vi "总磷氨氮通讯.vi"() -> ()   [LabVIEW 2016, in "CodCr.lvlib"]
uses:
  CodCr.lvlib
  <vilib>/Plasmionique/MB Master/MB_Master_Serial/MB_Master_Serial.lvclass
  <vilib>/Utility/config.llb/NI_LVConfig.lvlib
  <vilib>/Plasmionique/MB Master/MB_Master/MB_Master.lvclass
  <vilib>/Plasmionique/MB Master/MB Master.lvlib
  <vilib>/ptbypt/NI_PtbyPt.lvlib
  <vilib>/Utility/config.llb/Write Key (String).vi
  <vilib>/Utility/config.llb/Read Key (String).vi
  <vilib>/Utility/config.llb/Write Key (Boolean).vi
  <vilib>/Utility/config.llb/Read Key (Boolean).vi
  F:/Program Files/National Instruments/LabVIEW 2016/vi.lib/Plasmionique/MB Master/MB_Master/MB_Master.lvclass
panel:
  out "序列号":string
  out "状态告警区":T1
  out "测量数据区":T2 {"单位" items=["ug/L", "mg/L", "ppm", "mg/m3", "cm", "ppb", "ug/m3", "%", "nmol/mol", "umol/mol", "MPN/L", "MPN/100ml", "ng/m3", "NTU", "无量纲", "ms/cm", "us/cm", "℃", "mV", "万个/L"]}
  out "status":bool
  out "关键参数区":T3
  in  "读关键参数区":bool
  in  "读状态告警区":bool
  in  "读测量数据区":bool
  in  "站号":u16(ring) items=["总磷"=1, "氨氮"=3]
  in  "停止":bool
  in  "启动":bool
  in  "控制命令":u16(ring) items=["启动测量"=1, "标样核查"=2, "零点核查"=3, "跨度核查"=4, "空白测试"=5, "平行样测试"=6, "加标回收"=7, "空白校准"=8, "标样校准"=9, "初始化（清洗）"=10, "停止测试"=11, "仪器重启"=12, "校时"=13, "模式设置"=14, "测量间隔设置"=15]
  in  "控制命令参数":u16[](array[numeric]) format="%04xH"
  in  "VISA Resource":refnum<visa-resource-name>="COM16"
  in  "启用模块":bool
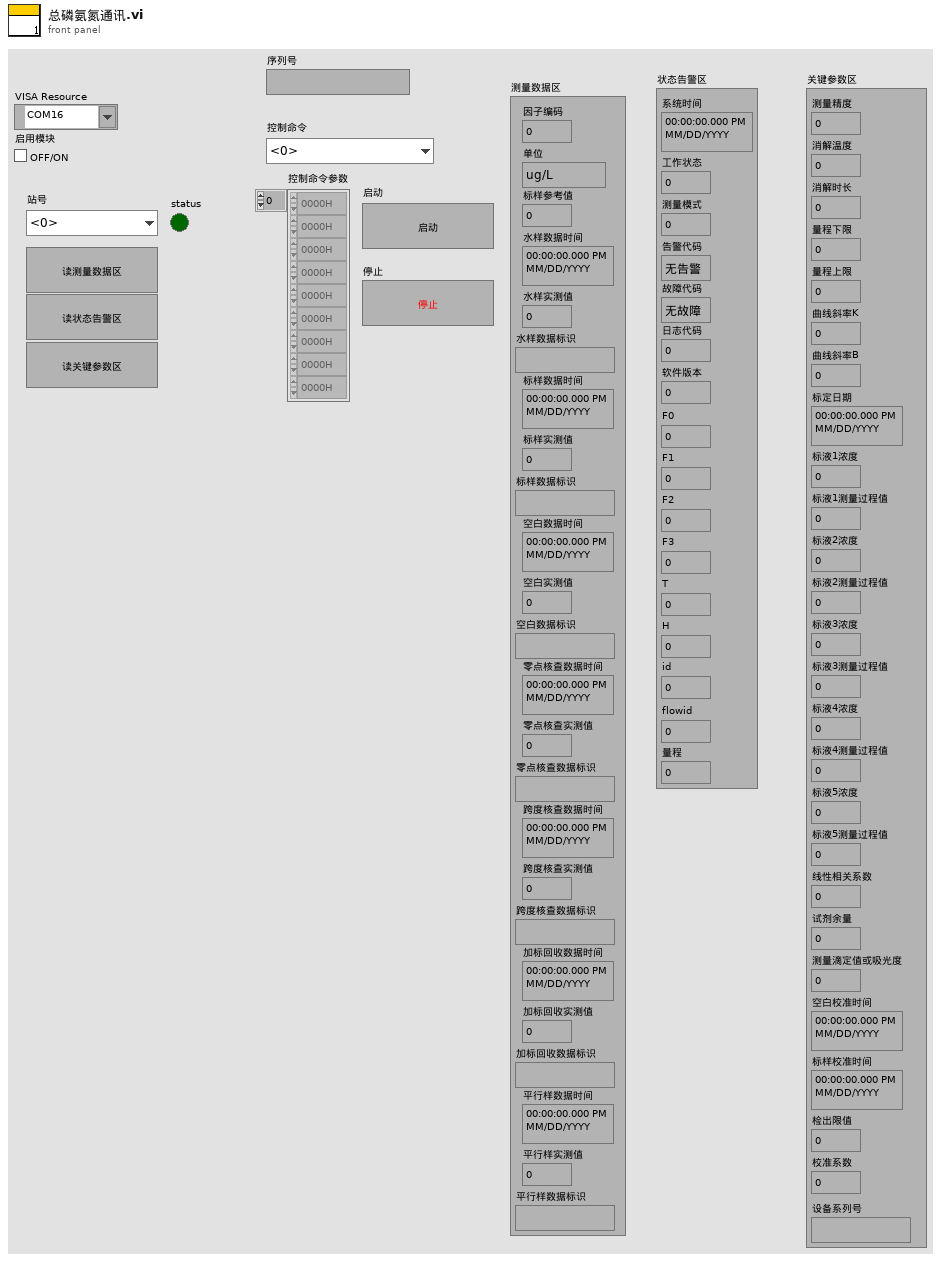
[diagram p1: front panel]
types:
  T1 = cluster{"系统时间":timestamp, "工作状态":u16, "测量模式":u16, "告警代码":enum16{"无告警", "缺试剂告警", "缺水样告警", "缺蒸馏水告警", "缺标液告警", "仪表漏液告警", "标定异常告警", "超量程告警", "加热异常", "低试剂预警", "超上限告警", "超下限告警", "仪表内部其他异常", "滴定异常告警", "电极异常告警", "量程切换告警", "参数设置告警", "PH电极电位异常", "电导率电极异常", "浊度光度异常", "溶解氧电极异常", "溶解氧光强异常", "温度异常告警", "PH异常告警", "溶解氧异常告警", "电导率异常告警", "浊度异常告警", "叶绿素异常告警", "藻密度异常告警", "蓝绿藻异常告警", "ORP异常告警", "氨氮异常告警", "清洁刷异常告警", "SD卡异常告警", "蓝牙异常告警", "Wifi异常告警", "流程异常告警"}, "故障代码":enum16{"无故障", "电机故障", "温度故障", "通讯故障", "滴定故障"}, "日志代码":u16, "软件版本":u16, "F0":sgl, "F1":sgl, "F2":sgl, "F3":sgl, "T":sgl, "H":sgl, "id":u16, "flowid":u16, "量程":u16}
  T2 = cluster{"因子编码":u32, "单位":u16, "标样参考值":sgl, "水样数据时间":timestamp, "水样实测值":sgl, "水样数据标识":string, "标样数据时间":timestamp, "标样实测值":sgl, "标样数据标识":string, "空白数据时间":timestamp, "空白实测值":sgl, "空白数据标识":string, "零点核查数据时间":timestamp, "零点核查实测值":sgl, "零点核查数据标识":string, "跨度核查数据时间":timestamp, "跨度核查实测值":sgl, "跨度核查数据标识":string, "加标回收数据时间":timestamp, "加标回收实测值":sgl, "加标回收数据标识":string, "平行样数据时间":timestamp, "平行样实测值":sgl, "平行样数据标识":string}
  T3 = cluster{"测量精度":u16, "消解温度":u16, "消解时长":u16, "量程下限":sgl, "量程上限":sgl, "曲线斜率K":sgl, "曲线斜率B":sgl, "标定日期":timestamp, "标液1浓度":sgl, "标液1测量过程值":sgl, "标液2浓度":sgl, "标液2测量过程值":sgl, "标液3浓度":sgl, "标液3测量过程值":sgl, "标液4浓度":sgl, "标液4测量过程值":sgl, "标液5浓度":sgl, "标液5测量过程值":sgl, "线性相关系数":sgl, "试剂余量":u32, "测量滴定值或吸光度":sgl, "空白校准时间":timestamp, "标样校准时间":timestamp, "检出限值":sgl, "校准系数":sgl, "设备系列号":string}
  T4 = typedef "NI_LVConfig.lvlib/Config Data RefNum.ctl" = refnum<k1>
  T5 = enum8{"Enabled", "Disabled", "Disabled and Grayed Out"}
  T6 = cluster{"baud rate (bps)":u32, "stop bits":u16, "parity":u16, "flow control":u16, "timeout":u32, "retries":i32}
  T7 = cluster{"因子编码":u32, "单位":u16, "标样参考值":sgl, "水样数据时间":timestamp, "水样实测值":sgl, "水样数据标识":string, "标样数据时间":timestamp, "标样实测值":sgl, "标样数据标识":string, "空白数据时间":timestamp, "空白实测值":sgl, "空白数据标识":string, "零点核查数据时间":timestamp, "零点核查实测值":sgl, "零点核查数据标识":string, "跨度核查数据时间":timestamp, "跨度核查实测值":sgl, "跨度核查数据标识":string, "加标回收数据时间":timestamp, "加标回收实测值":sgl, "加标回收数据标识":string, "平行样数据时间":timestamp, "平行样实测值":sgl, "平行样数据标识":string, "F0":sgl, "F1":sgl, "F2":sgl, "F3":sgl, "F4":sgl, "F5":sgl, "F6":sgl, "F7":sgl, "温度":sgl, "湿度":sgl, "X值":sgl}
  T8 = cluster{"系统时间":timestamp, "工作状态":enum16{"空闲", "水样测试", "标样核查", "零点核查", "跨度核查", "空白测试", "平行样测试", "加标回收", "空白校准", "标样校准", "初始化（清洗）"}, "测量模式":enum16{"待机", "连续模式", "周期模式", "定点模式", "受控模式", "手动模式"}, "告警代码":enum16{"无告警", "缺试剂告警", "缺水样告警", "缺蒸馏水告警", "缺标液告警", "仪表漏液告警", "标定异常告警", "超量程告警", "加热异常", "低试剂预警", "超上限告警", "超下限告警", "仪表内部其他异常", "滴定异常告警", "电极异常告警", "量程切换告警", "参数设置告警", "PH电极电位异常", "电导率电极异常", "浊度光度异常", "溶解氧电极异常", "溶解氧光强异常", "温度异常告警", "PH异常告警", "溶解氧异常告警", "电导率异常告警", "浊度异常告警", "叶绿素异常告警", "藻密度异常告警", "蓝绿藻异常告警", "ORP异常告警", "氨氮异常告警", "清洁刷异常告警", "SD卡异常告警", "蓝牙异常告警", "Wifi异常告警", "流程异常告警"}, "故障代码":enum16{"无故障", "电机故障", "温度故障", "通讯故障", "滴定故障"}, "日志代码":u16, "软件版本":u16, "F0":sgl, "F1":sgl, "F2":sgl, "F3":sgl, "T":sgl, "H":sgl, "id":u16, "flowid":u16, "量程":u16, "总磷控温温度1":sgl, "营养盐控温温度2":sgl, "ADC":sgl}
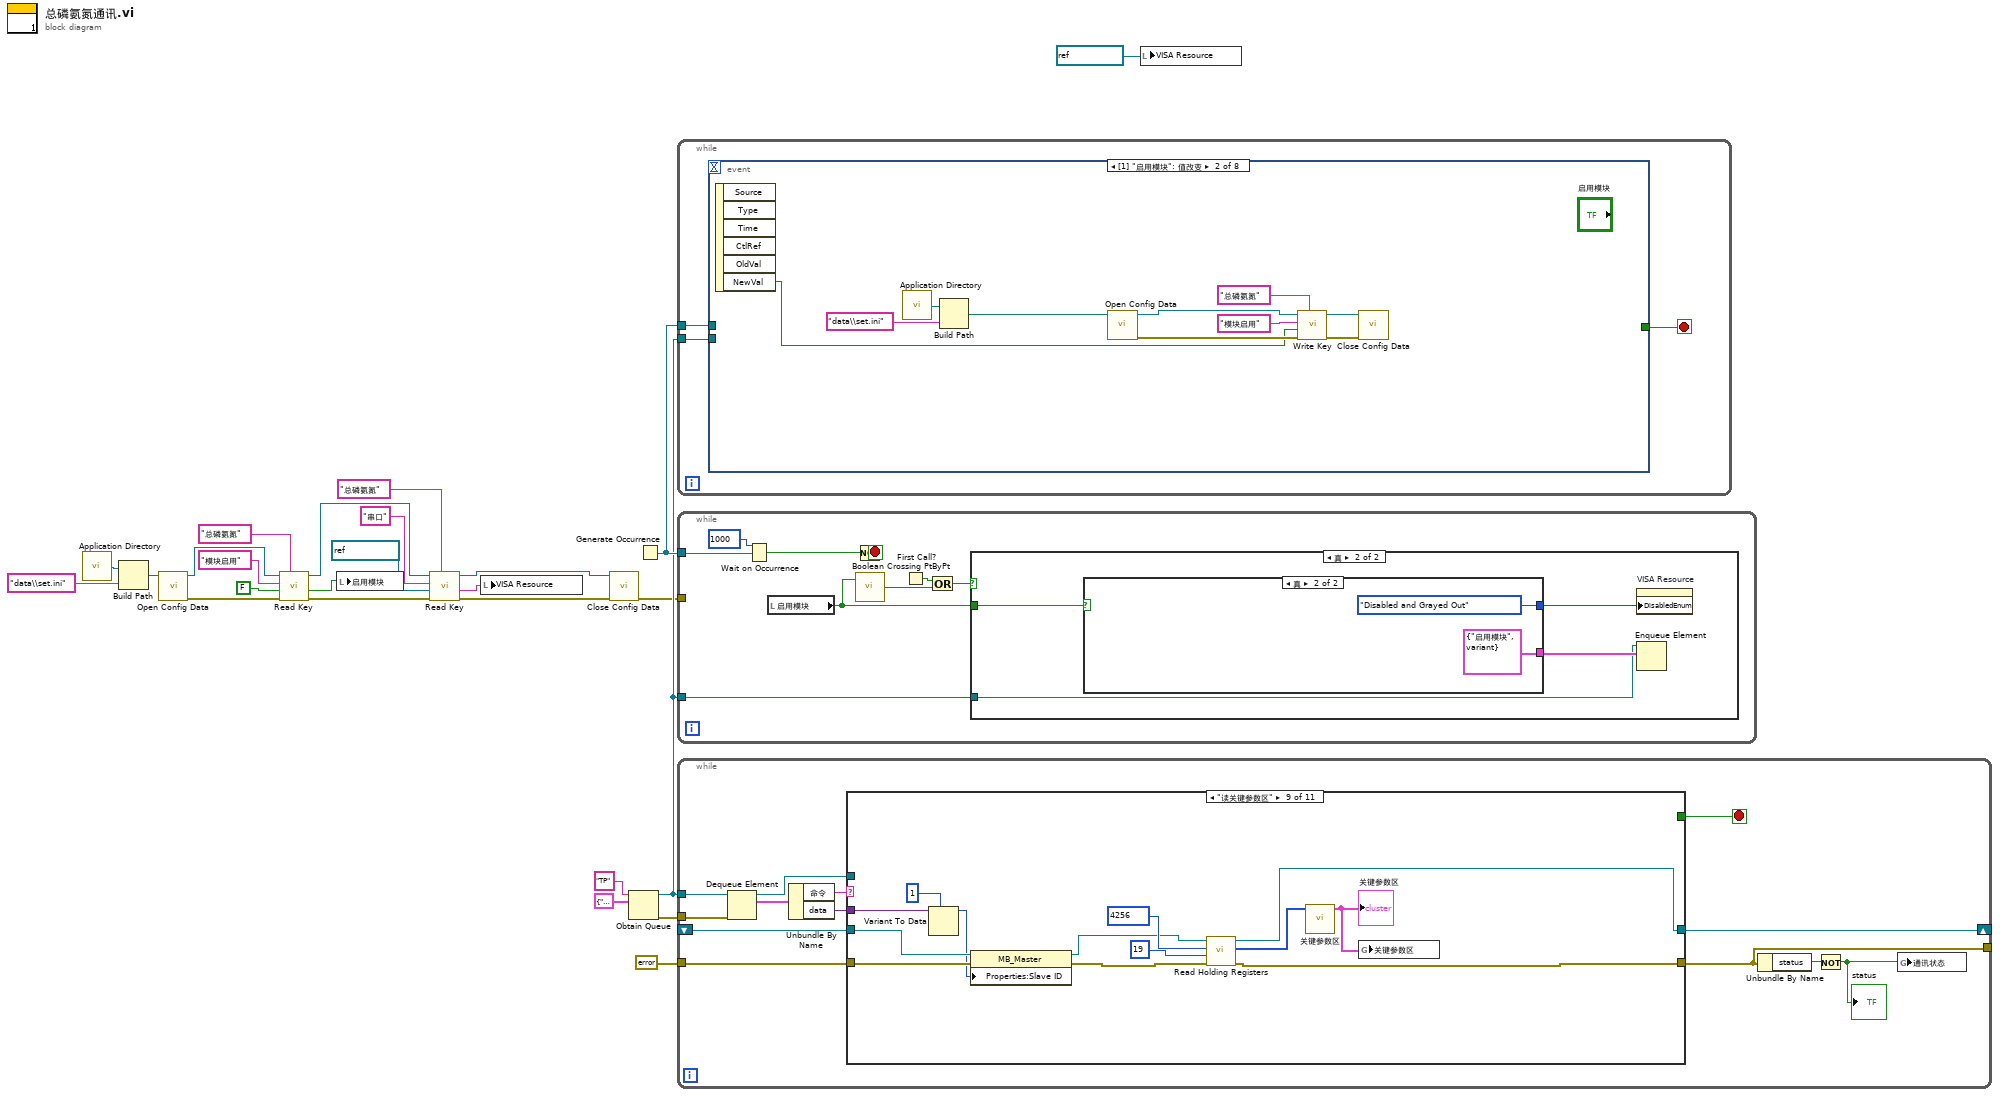
[diagram p0: block diagram]
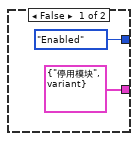
[diagram p3: hidden frame]
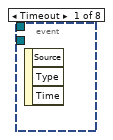
[diagram p4: hidden frame]
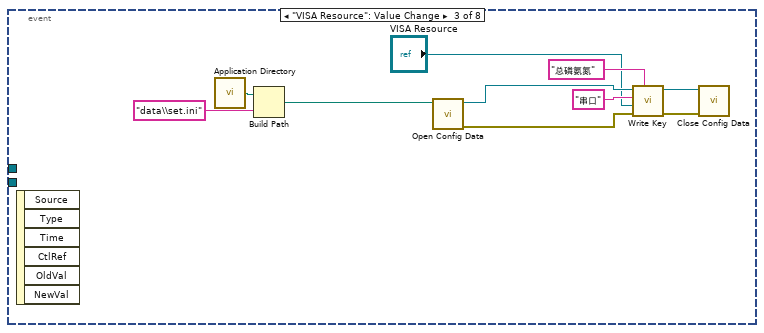
[diagram p5: hidden frame]
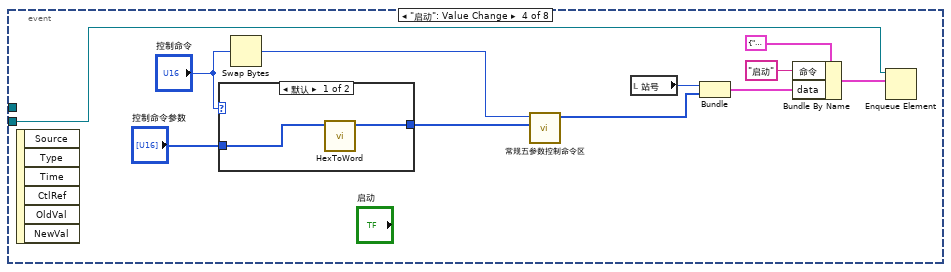
[diagram p6: hidden frame]
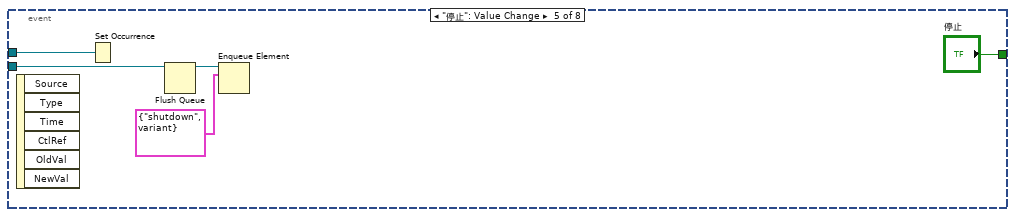
[diagram p8: hidden frame]
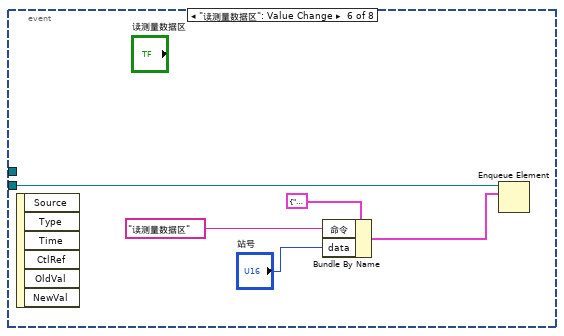
[diagram p9: hidden frame]
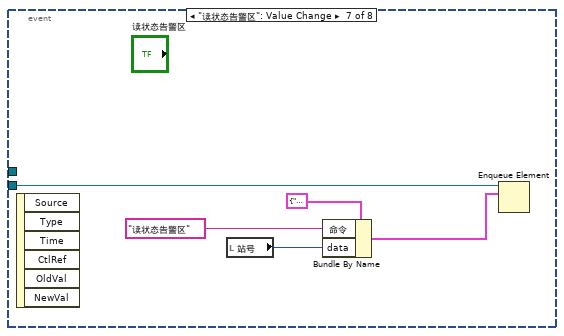
[diagram p10: hidden frame]
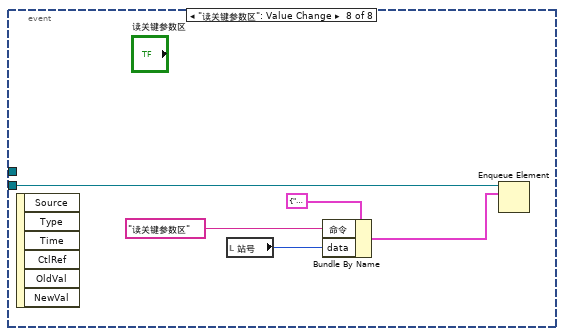
[diagram p11: hidden frame]
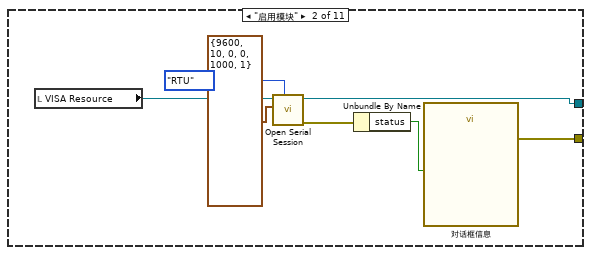
[diagram p13: hidden frame]
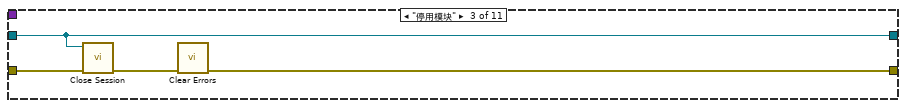
[diagram p14: hidden frame]
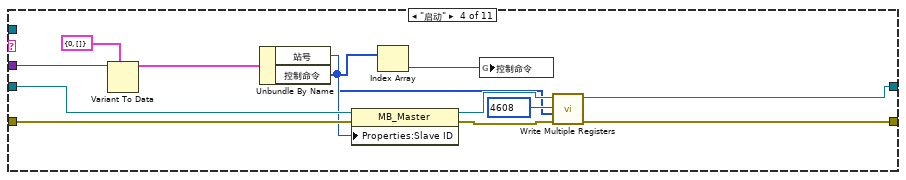
[diagram p15: hidden frame]
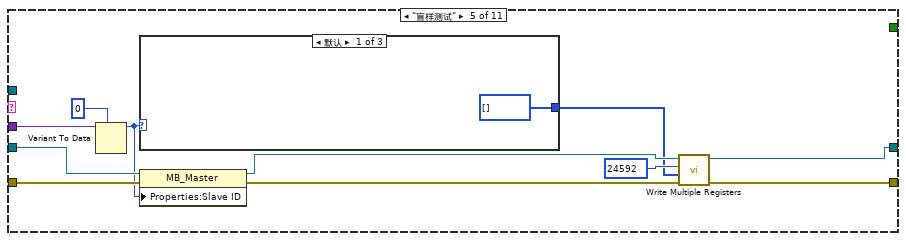
[diagram p16: hidden frame]
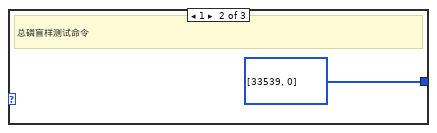
[diagram p17: hidden frame]
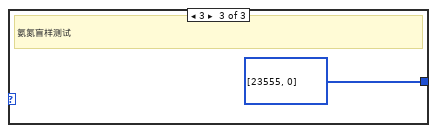
[diagram p18: hidden frame]
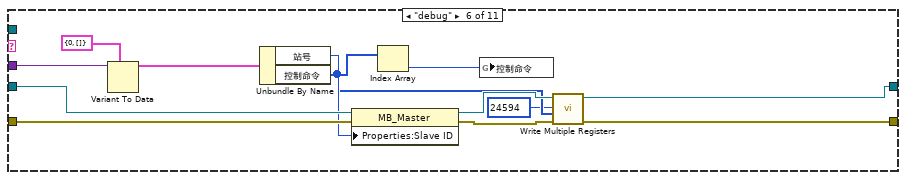
[diagram p19: hidden frame]
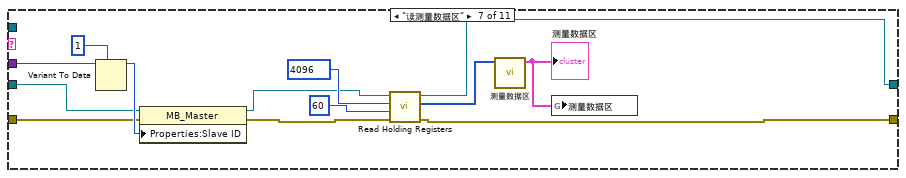
[diagram p20: hidden frame]
diagram:
  n1 = call <vilib>:"Application Directory.vi"() -> ("Application Directory"=w13:path)
  n2 = Build Path(base path=w13, name or relative path="data\\set.ini" ("名称或相对路径")) -> (appended path=w14:path)
  n3 = call <vilib>:"Open Config Data.vi"("configuration file path"=w14) -> ("error out"=w19:errorcluster, "refnum"=w18:T4)  [unwired: 8 in, 1 out]
  n4 = call-poly <vilib>:"Read Key.vi"("section"="总磷氨氮", "error in (no error)"=w19, "default value"=FALSE ("启用模块"), "key"="模块启用", "refnum"=w18) -> ("error out"=w7:errorcluster, "value"=w10:bool, "refnum out"=w9:T4)  [unwired: 3 in, 1 out]
  n5 = local write "启用模块"(w10) -> ()
  n6 = call-poly <vilib>:"Read Key.vi"("section"="总磷氨氮", "error in (no error)"=w7, "default value"=refnum<visa-resource-name> "COM16" ("VISA Resource"), "key"="串口", "refnum"=w9) -> ("error out"=w6:errorcluster, "value"=w3:string, "refnum out"=w8:T4)  [unwired: 3 in, 1 out]
  n7 = local write "VISA Resource"(w3) -> ()
  n8 = call <vilib>:"Close Config Data.vi"("error in (no error)"=w6, "refnum"=w8) -> ("error out"=w11:errorcluster)  [unwired: 8 in, 1 out]
  n9 = Obtain Queue(name (unnamed)="TP" ("名称（未命名）"), element data type=cluster{"命令":string, "data":variant} {"命令"="", "data"=variant}) -> (queue out=w20:refnum<queue>, error out=w23:errorcluster)  [unwired: 3 in, 1 out]
  n10 = Generate Occurrence() -> (w21:refnum<k4>)
  n11 = while {
    tunnel: w20 -> [w28]
    tunnel: w21 -> [w26]
    stop <- w27 stop-if-true
    n12 = event shown="[1] \"启用模块\": 值改变" {
      selector: _ -> [_ _ _ _ _ _ _ _]
      dyn-events: _ -> [_ _ _ _ _ _ _ _]
      timeout: _ -> [_ _ _ _ _ _ _ _]
      tunnel: w28 -> [_ _ _ w59 w66 w72 w77 w82]
      tunnel: [_ _ _ _ "停止" _ _ _] -> w27
      tunnel: w26 -> [_ _ _ _ w63 _ _ _]
      event Timeout {
        n13 = event-data() -> ()  [unwired: 1 in, 3 out]
      }
      event "启用模块": Value Change {
        n14 = event-data() -> ("NewVal"=w29:bool)  [unwired: 1 in, 5 out]
        n15 = call <vilib>:"Application Directory.vi"() -> ("Application Directory"=w31:path)
        n16 = Build Path(base path=w31, name or relative path="data\\set.ini" ("名称或相对路径")) -> (appended path=w32:path)
        n17 = call <vilib>:"Open Config Data.vi"("configuration file path"=w32) -> ("error out"=w38:errorcluster, "refnum"=w37:T4)  [unwired: 8 in, 1 out]
        n18 = call-poly <vilib>:"Write Key.vi"("section"="总磷氨氮", "error in (no error)"=w38, "value"=w29, "key"="模块启用", "refnum"=w37) -> ("error out"=w34:errorcluster, "refnum out"=w30:T4)  [unwired: 4 in, 1 out]
        n19 = call <vilib>:"Close Config Data.vi"("error in (no error)"=w34, "refnum"=w30) -> ()  [unwired: 8 in, 2 out]
      }
      event "VISA Resource": Value Change {
        n20 = event-data() -> ()  [unwired: 1 in, 6 out]
        n21 = call <vilib>:"Application Directory.vi"() -> ("Application Directory"=w41:path)
        n22 = Build Path(base path=w41, name or relative path="data\\set.ini" ("名称或相对路径")) -> (appended path=w42:path)
        n23 = call <vilib>:"Open Config Data.vi"("configuration file path"=w42) -> ("error out"=w48:errorcluster, "refnum"=w47:T4)  [unwired: 8 in, 1 out]
        n24 = call-poly <vilib>:"Write Key.vi"("section"="总磷氨氮", "error in (no error)"=w48, "value"="VISA Resource", "key"="串口", "refnum"=w47) -> ("error out"=w44:errorcluster, "refnum out"=w40:T4)  [unwired: 4 in, 1 out]
        n25 = call <vilib>:"Close Config Data.vi"("error in (no error)"=w44, "refnum"=w40) -> ()  [unwired: 8 in, 2 out]
      }
      event "启动": Value Change {
        n26 = event-data() -> ()  [unwired: 1 in, 6 out]
        n27 = case shown="默认" "控制命令" {
          tunnel: "控制命令参数" -> [w61 w62]
          tunnel: [w60 w62] -> w49
          frame Default {
            n28 = call "HexToWord.vi"("数组"=w61) -> ("WORD"=w60:u16[])  [unwired: 10 in]
          }
          frame 13 {
          }
        }
        n29 = Swap Bytes(anything="控制命令") -> (byte swapped=w52:u16)
        n30 = call "常规五参数控制命令区.vi"("控制命令参数"=w49, "控制命令"=w52) -> ("控制命令输出"=w55:u16[])  [unwired: 9 in]
        n31 = local read "站号"() -> (w54:u16)
        n32 = Bundle("站号"=w54, "控制命令输出"=w55) -> (w53:cluster{"站号":u16, "控制命令输出":u16[]})  [unwired: 1 in]
        n33 = Bundle By Name(cluster=cluster{"命令":string, "data":variant} {"命令"="", "data"=variant} ("元素"), "命令"="启动", "data"=w53) -> (w57:cluster{"命令":string, "data":variant})
        n34 = Enqueue Element(queue=w59, element=w57) -> ()  [unwired: 2 in, 3 out]
      }
      event "停止": Value Change {
        n35 = event-data() -> ()  [unwired: 1 in, 6 out]
        n36 = Set Occurrence(w63) -> ()
        n37 = Flush Queue(queue=w66) -> (queue out=w65:refnum<queue>)  [unwired: 1 in, 2 out]
        n38 = Enqueue Element(queue=w65, element=cluster{"命令":string, "data":variant} {"命令"="shutdown", "data"=variant} ("元素")) -> ()  [unwired: 2 in, 3 out]
      }
      event "读测量数据区": Value Change {
        n39 = event-data() -> ()  [unwired: 1 in, 6 out]
        n40 = Bundle By Name(cluster=cluster{"命令":string, "data":variant} {"命令"="", "data"=variant} ("元素"), "命令"="读测量数据区", "data"="站号") -> (w70:cluster{"命令":string, "data":variant})
        n41 = Enqueue Element(queue=w72, element=w70) -> ()  [unwired: 2 in, 3 out]
      }
      event "读状态告警区": Value Change {
        n42 = event-data() -> ()  [unwired: 1 in, 6 out]
        n43 = local read "站号"() -> (w73:u16)
        n44 = Bundle By Name(cluster=cluster{"命令":string, "data":variant} {"命令"="", "data"=variant} ("元素"), "命令"="读状态告警区", "data"=w73) -> (w75:cluster{"命令":string, "data":variant})
        n45 = Enqueue Element(queue=w77, element=w75) -> ()  [unwired: 2 in, 3 out]
      }
      event "读关键参数区": Value Change {
        n46 = event-data() -> ()  [unwired: 1 in, 6 out]
        n47 = local read "站号"() -> (w78:u16)
        n48 = Bundle By Name(cluster=cluster{"命令":string, "data":variant} {"命令"="", "data"=variant} ("元素"), "命令"="读关键参数区", "data"=w78) -> (w80:cluster{"命令":string, "data":variant})
        n49 = Enqueue Element(queue=w82, element=w80) -> ()  [unwired: 2 in, 3 out]
      }
    }
  }
  n50 = while {
    tunnel: w21 -> [w91]
    tunnel: w20 -> [w86]
    tunnel: w11 -> [_]
    stop <- w88 stop-if-true
    n51 = Wait on Occurrence(2:w91, 3:1000 ("毫秒超时(-1)")) -> (0:w89:bool)  [unwired: 1 in]
    n52 = local read "启用模块"() -> (w87:bool)
    n53 = Not(x=w89) -> (.not. x?=w88:bool)
    n54 = call <vilib>:"Boolean Crossing PtByPt.vi"("input"=w87) -> ("crossing"=w84:bool)  [unwired: 2 in]
    n55 = First Call?() -> (First Call?: T/F=w85:bool)
    n56 = Or(x=w85, y=w84) -> (x .or. y?=w83:bool)
    n57 = case shown="真" w83 {
      tunnel: w87 -> [_ w94]
      tunnel: w86 -> [_ w93]
      frame False {
      }
      frame True {
        n58 = case shown="真" w94 {
          tunnel: [cluster{"命令":string, "data":variant} {"命令"="停用模块", "data"=variant} ("元素") cluster{"命令":string, "data":variant} {"命令"="启用模块", "data"=variant} ("元素")] -> w95
          tunnel: [T5."Enabled" ("禁用") T5."Disabled and Grayed Out" ("禁用")] -> w92
          frame False {
          }
          frame True {
          }
        }
        n59 = property on="VISA Resource" class="VISAName"("DisabledEnum"=w92) -> ()  [unwired: 2 in, 2 out]
        n60 = Enqueue Element(queue=w93, element=w95) -> ()  [unwired: 2 in, 3 out]
      }
    }
  }
  n61 = while {
    tunnel: w20 -> [w112]
    tunnel: w23 -> [w111]
    shift-right: [w109] -> _
    shift-left: _ -> [w108]
    tunnel: errorcluster {"status"=FALSE, "code"=0, "source"=""} ("error out") -> [w107]
    tunnel: [w102] -> _
    stop <- w110 stop-if-true
    n62 = Dequeue Element(queue=w112, error in (no error)=w111) -> (queue out=w103:refnum<queue>, element=w105:cluster{"命令":string, "data":variant})  [unwired: 1 in, 2 out]
    n63 = Unbundle By Name(w105) -> ("命令"=w106:string, "data"=w104:variant)
    n64 = case shown="\"读关键参数区\"" w106 {
      tunnel: w104 -> [_ _ _ w135 w146 w163 w172 w181 w196 w210 _]
      tunnel: w103 -> [_ _ _ _ _ _ _ _ _ _ w223]
      tunnel: [_ _ _ _ _ _ _ _ _ _ TRUE] -> w110
      tunnel: [w113 w121 w122 w138 w149 w165 w177 w190 w203 w217 w219] -> w109
      tunnel: [w114 w116 w123 w137 w148 w164 w178 w191 w204 w218 w220] -> w102
      tunnel: w108 -> [w113 _ w122 w134 w145 w162 w171 w184 w199 w213 w219]
      tunnel: w107 -> [w114 _ w125 w131 w142 w159 w169 w185 w200 w214 w221]
      frame Default {
      }
      frame "启用模块" {
        n65 = local read "VISA Resource"() -> (w115:refnum<visa-resource-name>)
        n66 = call <vilib>:"Open Serial Session.vi"("Mode (RTU)"=enum16{"RTU", "ASCII"}."RTU", "Serial Config"=T6 {"baud rate (bps)"=9600, "stop bits"=10, "parity"=0, "flow control"=0, "timeout"=1000, "retries"=1}, "VISA Resource"=w115) -> ("Error out"=w117:errorcluster, "MB_Serial session"=w121:refnum<class "MB_Master_Serial.lvclass">)  [unwired: 7 in]
        n67 = Unbundle By Name(w117) -> ("status"=w118:bool)
        n68 = call "对话框信息"("Enable"=w118) -> ("error out"=w116:errorcluster)  [unwired: 9 in, 1 out]
      }
      frame "停用模块" {
        n69 = call-dynamic "Close Session.vi"("error in (no error)"=w125, "MB session in"=w122) -> ("error out"=w124:errorcluster)  [unwired: 9 in]
        n70 = call <vilib>:"Clear Errors.vi"("error in (no error)"=w124) -> ("error out"=w123:errorcluster)  [unwired: 5 in, 1 out]
      }
      frame "启动" {
        n71 = Variant To Data(type=cluster{"站号":u16, "控制命令":u16[]} {"站号"=0, "控制命令"=[]} ("输出簇"), Variant=w135) -> (data=w129:cluster{"站号":u16, "控制命令":u16[]})  [unwired: 1 in, 1 out]
        n72 = Unbundle By Name(w129) -> ("站号"=w128:u16, "控制命令"=w126:u16[])
        n73 = property class="MB_Master"(reference=w134, error in=w131, "Properties:Slave ID"=w128) -> (reference out=w133:refnum<class "MB_Master.lvclass">, error out=w132:errorcluster)
        n74 = Index Array(array=w126) -> (element=w127:u16)  [unwired: 1 in]
        n75 = global write "VAR总磷总氮全局变量.vi" "控制命令"(w127) -> ()
        n76 = call <vilib>:"Write Multiple Registers.vi"("error in (no error)"=w132, "values"=w126, "starting address"=u16 4608, "MB session in"=w133) -> ("error out"=w137:errorcluster, "MB session out"=w138:refnum<class "MB_Master.lvclass">)  [unwired: 6 in]
      }
      frame "盲样测试" {
        n77 = Variant To Data(type=0, Variant=w146) -> (data=w139:i32)  [unwired: 1 in, 1 out]
        n78 = case shown="默认" w139 {
          tunnel: [u16[] [] ("values") u16[] [33539, 0] ("values") u16[] [23555, 0] ("values")] -> w141
          frame Default {
          }
          frame 1 {
            # "总磷盲样测试命令"
          }
          frame 3 {
            # "氨氮盲样测试"
          }
        }
        n79 = property class="MB_Master"(reference=w145, error in=w142, "Properties:Slave ID"=w139) -> (reference out=w144:refnum<class "MB_Master.lvclass">, error out=w143:errorcluster)
        n80 = call <vilib>:"Write Multiple Registers.vi"("error in (no error)"=w143, "values"=w141, "starting address"=u16 24592, "MB session in"=w144) -> ("error out"=w148:errorcluster, "MB session out"=w149:refnum<class "MB_Master.lvclass">)  [unwired: 6 in]
      }
      frame "debug" {
        n81 = Variant To Data(type=cluster{"站号":u16, "控制命令":u16[]} {"站号"=0, "控制命令"=[]} ("输出簇"), Variant=w163) -> (data=w157:cluster{"站号":u16, "控制命令":u16[]})  [unwired: 1 in, 1 out]
        n82 = Unbundle By Name(w157) -> ("站号"=w156:u16, "控制命令"=w154:u16[])
        n83 = property class="MB_Master"(reference=w162, error in=w159, "Properties:Slave ID"=w156) -> (reference out=w161:refnum<class "MB_Master.lvclass">, error out=w160:errorcluster)
        n84 = Index Array(array=w154) -> (element=w155:u16)  [unwired: 1 in]
        n85 = global write "VAR总磷总氮全局变量.vi" "控制命令"(w155) -> ()
        n86 = call <vilib>:"Write Multiple Registers.vi"("error in (no error)"=w160, "values"=w154, "starting address"=u16 24594, "MB session in"=w161) -> ("error out"=w164:errorcluster, "MB session out"=w165:refnum<class "MB_Master.lvclass">)  [unwired: 6 in]
      }
      frame "读测量数据区" {
        n87 = Variant To Data(type=u8 1 ("Slave ID"), Variant=w172) -> (data=w173:u8)  [unwired: 1 in, 1 out]
        n88 = property class="MB_Master"(reference=w171, error in=w169, "Properties:Slave ID"=w173) -> (reference out=w170:refnum<class "MB_Master.lvclass">, error out=w168:errorcluster)
        n89 = call <vilib>:"Read Holding Registers.vi"("error in (no error)"=w168, "quantity"=u16 60, "starting address"=u16 4096, "MB session in"=w170) -> ("error out"=w178:errorcluster, "Registers"=w167:u16[], "MB session out"=w177:refnum<class "MB_Master.lvclass">)  [unwired: 5 in]
        n90 = call "测量数据区.vi"("数组"=w167) -> ("测量数据区"=w166:T7)  [unwired: 10 in]
        "测量数据区" <- w166
        n91 = global write "VAR总磷总氮全局变量.vi" "测量数据区"(w166) -> ()
      }
      frame "读状态告警区" {
        n92 = Variant To Data(type=u8 1 ("Slave ID"), Variant=w181) -> (data=w186:u8)  [unwired: 1 in, 1 out]
        n93 = property class="MB_Master"(reference=w184, error in=w185, "Properties:Slave ID"=w186) -> (reference out=w183:refnum<class "MB_Master.lvclass">, error out=w182:errorcluster)
        n94 = call <vilib>:"Read Holding Registers.vi"("error in (no error)"=w182, "quantity"=u16 24, "starting address"=u16 4224, "MB session in"=w183) -> ("error out"=w191:errorcluster, "Registers"=w180:u16[], "MB session out"=w190:refnum<class "MB_Master.lvclass">)  [unwired: 5 in]
        n95 = call "状态告警区.vi"("数组"=w180) -> ("状态告警区"=w179:T8)  [unwired: 10 in]
        "状态告警区" <- w179
        n96 = global write "VAR总磷总氮全局变量.vi" "状态告警区"(w179) -> ()
      }
      frame "读关键参数区" {
        n97 = Variant To Data(type=u8 1 ("Slave ID"), Variant=w196) -> (data=w194:u8)  [unwired: 1 in, 1 out]
        n98 = property class="MB_Master"(reference=w199, error in=w200, "Properties:Slave ID"=w194) -> (reference out=w198:refnum<class "MB_Master.lvclass">, error out=w197:errorcluster)
        n99 = call <vilib>:"Read Holding Registers.vi"("error in (no error)"=w197, "quantity"=u16 19, "starting address"=u16 4256, "MB session in"=w198) -> ("error out"=w204:errorcluster, "Registers"=w193:u16[], "MB session out"=w203:refnum<class "MB_Master.lvclass">)  [unwired: 5 in]
        n100 = call "关键参数区.vi"("数组"=w193) -> ("关键参数区"=w192:T3)  [unwired: 10 in]
        "关键参数区" <- w192
        n101 = global write "VAR总磷总氮全局变量.vi" "关键参数区"(w192) -> ()
      }
      frame "读序列号" {
        n102 = Variant To Data(type=u8 1 ("Slave ID"), Variant=w210) -> (data=w208:u8)  [unwired: 1 in, 1 out]
        n103 = property class="MB_Master"(reference=w213, error in=w214, "Properties:Slave ID"=w208) -> (reference out=w212:refnum<class "MB_Master.lvclass">, error out=w211:errorcluster)
        n104 = call <vilib>:"Read Holding Registers.vi"("error in (no error)"=w211, "quantity"=u16 6, "starting address"=u16 3, "MB session in"=w212) -> ("error out"=w218:errorcluster, "Registers"=w207:u16[], "MB session out"=w217:refnum<class "MB_Master.lvclass">)  [unwired: 5 in]
        n105 = call "HexToString.vi"("数组"=w207) -> ("STRING"=w206:string[])  [unwired: 10 in]
        n106 = Index Array(array=w206) -> (element=w205:string)  [unwired: 1 in]
        "序列号" <- w205
        n107 = global write "VAR总磷总氮全局变量.vi" "序列号"(w205) -> ()
      }
      frame "shutdown" {
        n108 = call-dynamic "Close Session.vi"("error in (no error)"=w221, "MB session in"=w219) -> ("error out"=w220:errorcluster)  [unwired: 9 in]
        n109 = Flush Queue(queue=w223) -> (queue out=w222:refnum<queue>)  [unwired: 1 in, 2 out]
        n110 = Release Queue(queue=w222) -> ()  [unwired: 2 in, 3 out]
      }
    }
    n111 = Unbundle By Name(w102) -> ("status"=w101:bool)
    n112 = Not(x=w101) -> (.not. x?=w100:bool)
    "status" <- w100
    n113 = global write "VAR总磷总氮全局变量.vi" "通讯状态"(w100) -> ()
  }
  n114 = local write "VISA Resource"(refnum<visa-resource-name> "COM16" ("VISA Resource")) -> ()
